vi "create_project_vipc.vi"(6 "quiet? (T)":bool=TRUE, 8 "error in (no error)":errorcluster, 10 "dependencies_folder":path, 11 "project_file":path) -> (0 "error out":errorcluster)   [LabVIEW 2015, in "lv-build.lvlib"]
uses:
  lv-build.lvlib
  <vilib>/JKI/VIPM API/VIPM API_vipm_api.lvlib
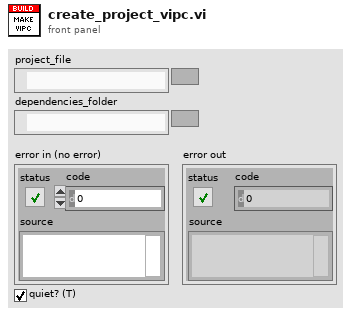
[diagram p1: front panel]
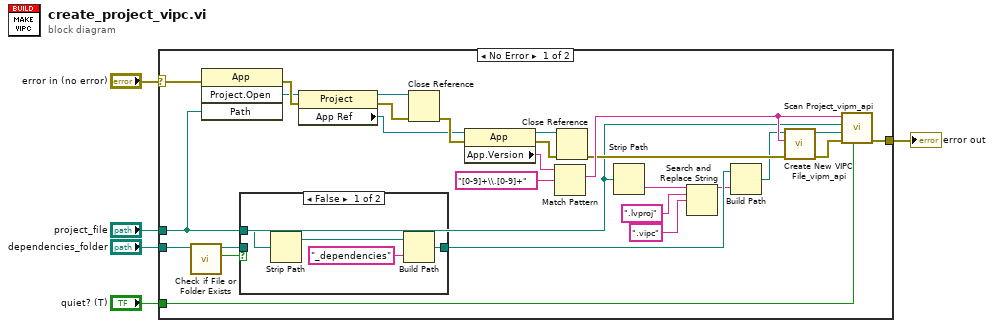
[diagram p0: block diagram]
diagram:
  n1 = case shown="No Error" "error in (no error)" {
    selector: "error in (no error)" -> [w19 w37]
    tunnel: "project_file" -> [w10 _]
    tunnel: [w26 w37] -> w3
    tunnel: "quiet? (T)" -> [w25 _]
    tunnel: "dependencies_folder" -> [w13 _]
    frame No Error {
      n2 = call <vilib>:"Check if File or Folder Exists.vi"("path"=w13) -> ("file or folder exists?"=w11:bool, "dup path"=w12:path)  [unwired: 8 in, 1 out]
      n3 = invoke class="App" method="Project.Open"(error in=w19, "Path"=w10) -> (error out=w29:errorcluster, "Project:Open"=w20:refnum<vi>)  [unwired: 2 in, 2 out]
      n4 = case shown="False" w11 {
        tunnel: [w34 w36] -> w14
        tunnel: w12 -> [_ w36]
        tunnel: w10 -> [w32 _]
        frame False {
          n5 = Strip Path(path=w32) -> (stripped path=w35:path)  [unwired: 1 out]
          n6 = Build Path(base path=w35, name or relative path="_dependencies") -> (appended path=w34:path)
        }
        frame True {
        }
      }
      n7 = property class="Project"(reference=w20, error in=w29) -> (reference out=w24:refnum<vi>, error out=w31:errorcluster, "App Ref"=w21:refnum<vi>)
      n8 = Close Reference(reference=w24, error in (no error)=w31) -> (error out=w30:errorcluster)
      n9 = property class="App"(reference=w21, error in=w30) -> (reference out=w22:refnum<vi>, error out=w23:errorcluster, "App.Version"=w18:string)
      n10 = Match Pattern(string=w18, regular expression="[0-9]+\\.[0-9]+") -> (match substring=w27:string)  [unwired: 1 in, 3 out]
      n11 = Close Reference(reference=w22, error in (no error)=w23) -> (error out=w16:errorcluster)
      n12 = Strip Path(path=w10) -> (name=w9:string)  [unwired: 1 out]
      n13 = Search and Replace String(input string=w9, search string=".lvproj" ("regular expression"), replace string=".vipc" ("string")) -> (result string=w8:string)  [unwired: 5 in, 3 out]
      n14 = Build Path(base path=w14, name or relative path=w8) -> (appended path=w15:path)
      n15 = call <vilib>:"Create New VIPC File_vipm_api.vi"("error in (no error)"=w16, "LabVIEW Version"=w27, "Path to New VIPC File"=w15) -> ("error out"=w17:errorcluster)  [unwired: 8 in]
      n16 = call <vilib>:"Scan Project_vipm_api.vi"("quiet? (T)"=w25, "error in (no error)"=w17, "Path to VIPC File"=w15, "Project file, VI or project dir path"=w10, "LabVIEW Version"=w27) -> ("error out"=w26:errorcluster)  [unwired: 6 in]
    }
    frame Error {
    }
  }
  "error out" <- w3
